vi "Manual Override Button Enable Disable Reactor.vi"(0 "Number of Shared Lines":i32, 2 "Reactor Number":i32, 3 "Valves Per Reactor":i32, 4 "Stop Program":refnum<vi>, 5 "Chamber Lock Claimed X":refnum<vi>, 6 "Pump Shared Lock Claimed Array":refnum<vi>, 7 "Manual Valve Array":refnum<vi>) -> ()   [LabVIEW 2022 SP3]
panel:
  out "Array":refnum<vi>[](array[refnum])
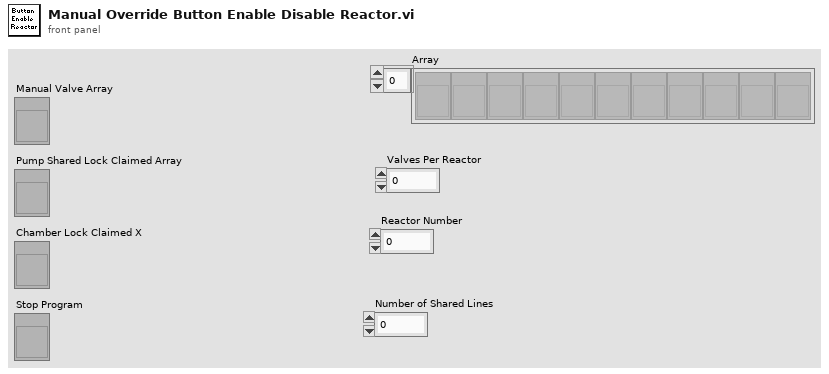
[diagram p1: front panel]
types:
  T1 = enum8{"Enabled", "Disabled", "Disabled and Grayed Out"}
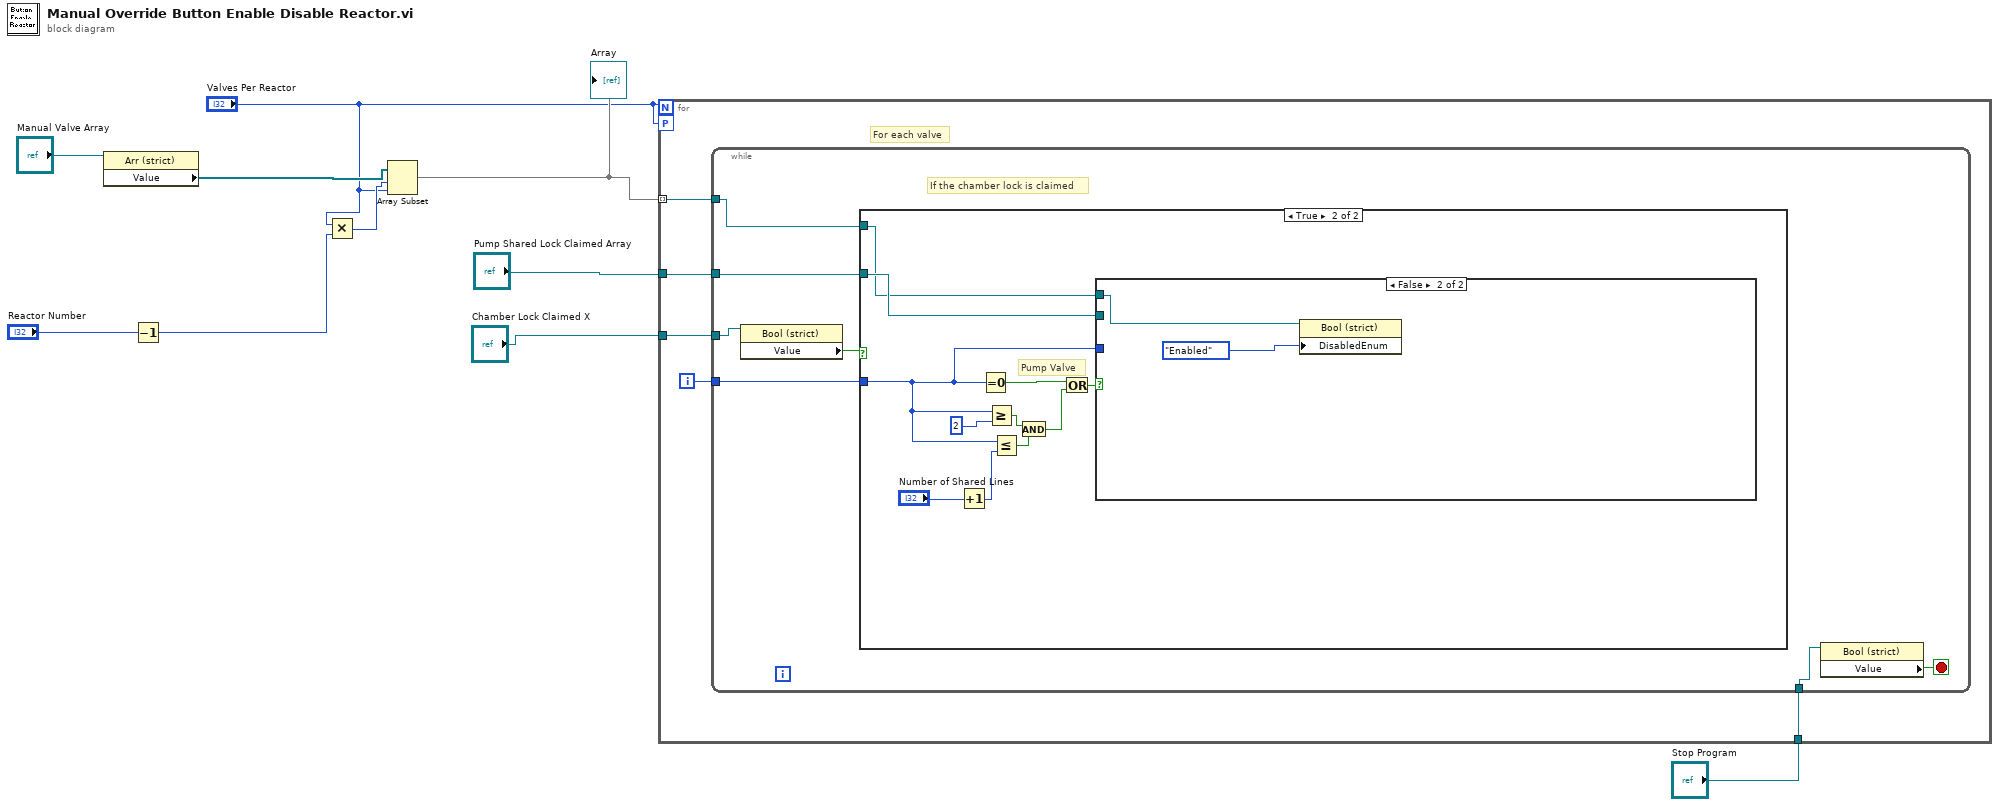
[diagram p0: block diagram]
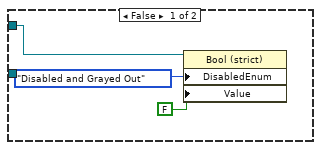
[diagram p2: hidden frame]
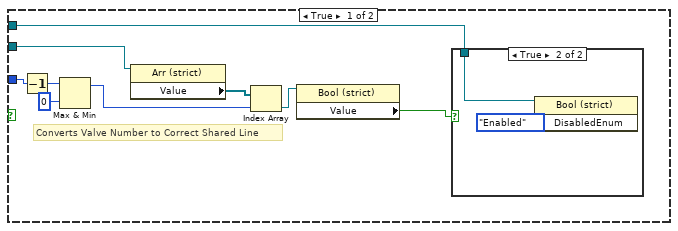
[diagram p3: hidden frame]
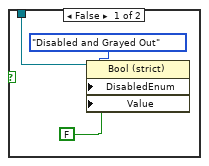
[diagram p4: hidden frame]
diagram:
  n1 = property class="Arr (strict)"(reference="Manual Valve Array") -> ("Value"=w5:refnum<vi>[])  [unwired: 1 in, 2 out]
  n2 = Decrement(x="Reactor Number") -> (x-1=w3:i32)
  n3 = Multiply(x="Valves Per Reactor", y=w3) -> (x*y=w2:i32)
  n4 = Array Subset(array=w5, index=w2, length="Valves Per Reactor") -> (w8:refnum<vi>[])
  "Array" <- w8
  n5 = for {
    N: "Valves Per Reactor" -> [_]
    workers-P: "Valves Per Reactor" -> [_]
    tunnel: "Pump Shared Lock Claimed Array" -> [w13]
    tunnel: w8 -> [w12] mode=indexing
    tunnel: "Stop Program" -> [w11]
    tunnel: "Chamber Lock Claimed X" -> [w14]
    i -> [w15]
    # "For each valve"
    n6 = while {
      tunnel: w15 -> [w22]
      tunnel: w14 -> [w20]
      tunnel: w13 -> [w19]
      tunnel: w12 -> [w18]
      tunnel: w11 -> [w16]
      stop <- w17 stop-if-true
      # "If the chamber lock is claimed"
      n7 = property class="Bool (strict)"(reference=w20) -> ("Value"=w21:bool)  [unwired: 1 in, 2 out]
      n8 = case shown="True" w21 {
        tunnel: w22 -> [_ w27]
        tunnel: w19 -> [_ w36]
        tunnel: w18 -> [w23 w35]
        frame False {
          n9 = property class="Bool (strict)"(reference=w23, "DisabledEnum"=T1."Disabled and Grayed Out" ("Disabled"), "Value"=FALSE) -> ()  [unwired: 1 in, 2 out]
        }
        frame True {
          # "Pump Valve"
          n10 = Increment(x="Number of Shared Lines") -> (x+1=w29:i32)
          n11 = Equal To 0?(x=w27) -> (x = 0?=w34:bool)
          n12 = Greater Or Equal?(x=w27, y=2) -> (x >= y?=w32:bool)
          n13 = Less Or Equal?(x=w27, y=w29) -> (x <= y?=w31:bool)
          n14 = And(x=w32, y=w31) -> (x .and. y?=w28:bool)
          n15 = Or(x=w34, y=w28) -> (x .or. y?=w26:bool)
          n16 = case shown="False" w26 {
            tunnel: w36 -> [w42 _]
            tunnel: w35 -> [w41 w51]
            tunnel: w27 -> [w40 _]
            frame True {
              # "Converts Valve Number to Correct Shared Line"
              n17 = Decrement(x=w40) -> (x-1=w39:i32)
              n18 = Max & Min(x=w39, y=0) -> (max(x,y)=w37:i32)  [unwired: 1 out]
              n19 = property class="Arr (strict)"(reference=w42) -> ("Value"=w45:refnum<vi>[])  [unwired: 1 in, 2 out]
              n20 = Index Array(array=w45, index=w37) -> (element=w44:refnum<vi>)
              n21 = property class="Bool (strict)"(reference=w44) -> ("Value"=w43:bool)  [unwired: 1 in, 2 out]
              n22 = case shown="True" w43 {
                tunnel: w41 -> [w46 w49]
                frame False {
                  n23 = property class="Bool (strict)"(reference=w46, "DisabledEnum"=T1."Disabled and Grayed Out" ("Disabled"), "Value"=FALSE) -> ()  [unwired: 1 in, 2 out]
                }
                frame True {
                  n24 = property class="Bool (strict)"(reference=w49, "DisabledEnum"=T1."Enabled" ("Disabled")) -> ()  [unwired: 1 in, 2 out]
                }
              }
            }
            frame False {
              n25 = property class="Bool (strict)"(reference=w51, "DisabledEnum"=T1."Enabled" ("Disabled")) -> ()  [unwired: 1 in, 2 out]
            }
          }
        }
      }
      n26 = property class="Bool (strict)"(reference=w16) -> ("Value"=w17:bool)  [unwired: 1 in, 2 out]
    }
  }
